vi "Chroma 1905x Series Preset Pass Hold Time.vi"(2 "error in":T1, 3 "Pass Time":dbl=0.6 min=0.2 max=99.9 step=0.1 format="%.1f", 4 "inst handle in":refnum<visa-resource-name>) -> (0 "error out":T1, 1 "inst handle out":refnum<visa-resource-name>)   [LabVIEW 2025]
doc: "Chroma\n5 Clock Tower Place Suite 210\nMaynard, MA 01754\nTel: 1 800 253-1230\nTel: 1 877 4 A HIPOT\nFax: 1 978-461-4295\nWebsite: www.chroma.com"
uses:
  <instrlib>/Chroma 19052/Chroma 19052.lvlib
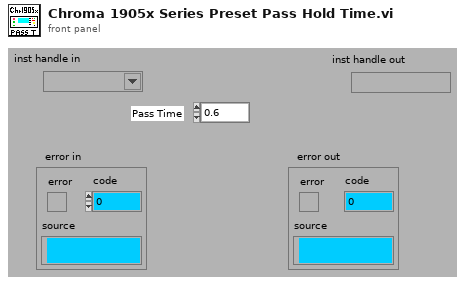
[diagram p1: front panel]
types:
  T1 = cluster{"error":bool, "code":i8, "source":string}
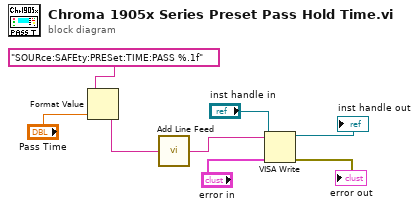
[diagram p0: block diagram]
diagram:
  n1 = Format Value(format string="SOURce:SAFEty:PRESet:TIME:PASS %.1f", value (0)="Pass Time") -> (output string=w2:string)  [unwired: 1 in]
  n2 = call <instrlib>:"Add Line Feed.vi"("Cmdstring"=w2) -> ("Concatenated String"=w1:string)
  n3 = VISA Write(VISA resource name="inst handle in", write buffer=w1, error in (no error)="error in") -> (VISA resource name out=→"inst handle out":refnum<visa-resource-name>, error out=→"error out":errorcluster)  [unwired: 1 out]
